vi "GetEvents.vi"(8 "error in (no error)":errorcluster, 11 "Camera in":refnum<class "Camera.lvclass">) -> (0 "error out":errorcluster, 2 "CameraEvents":T1, 3 "Camera out":refnum<class "Camera.lvclass">)   [LabVIEW 2020, in "CameraUSB.lvlib" / "Camera.lvclass"]
doc: "Return events generates from camera"
uses:
  Camera.lvclass
  ICamera/TypeDef/Events.ctl
  ICamera/TypeDef/StreamDataEvent.ctl
  Camera.lvclass/Camera.ctl
  ICamera/TypeDef/ICamera_typedef.lvlib
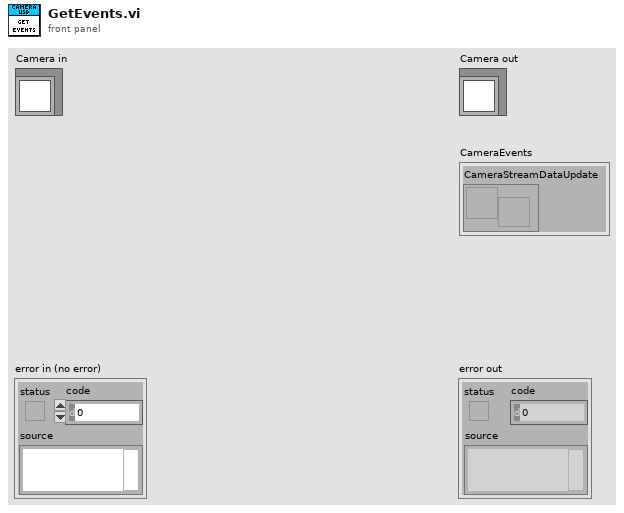
[diagram p1: front panel]
types:
  T1 = typedef "ICamera_typedef.lvlib/Events.ctl" = cluster{"CameraStreamDataUpdate":T2}
  T2 = typedef "ICamera_typedef.lvlib/StreamDataEvent.ctl" = refnum<user-event>
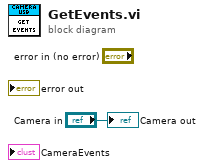
[diagram p0: block diagram]
diagram:
  "Camera out" <- "Camera in"
